vi "Device Test.vi"() -> ()   [LabVIEW 2011, in "Power Supply.lvclass"]
uses:
  Power Supply.lvclass
  Protection Limits.ctl
  Voltage Units.ctl
  Current Units.ctl
  Source Units.ctl
  Keithley 2400/Keithley 2400.lvclass
  Stanford Research PS350/Stanford Research PS350.lvclass
  Source Mode.ctl
panel:
  out "Source Value":dbl
  out "output":bool
  in  "Test":T1(ring)
  out "error out":errorcluster
  in  "Power Supply":enum16{"Keithley", "Stanford Research"}(ring)
  in  "Source Value Units":T2
  in  "Source Value":dbl=20.0
  in  "Limits":T3={"Voltage Limit"=100.0, "Voltage Limit Units"=enum."volts", "Current Limit"=1.0, "Current Limit Units"=enum."microamps", "Voltage Trip/Cmpl"=50.0, "Voltage Trip/Cmpl Units"=enum."volts", "Current Trip/Cmpl"=1.0, "Current Trip/Cmpl Units"=enum."microamps"}
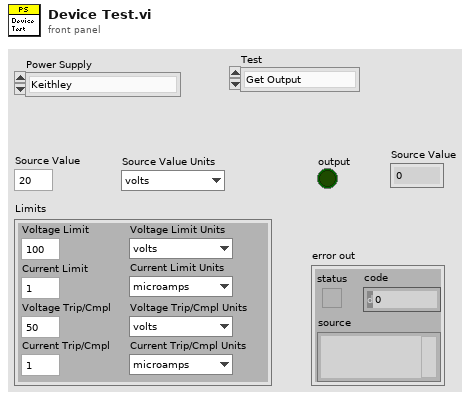
[diagram p1: front panel]
types:
  T1 = enum16{"Get Output", "Get Source Value", "Set Voltage"}
  T2 = typedef "Power Supply.lvclass/Source Units.ctl" = enum16{"volts", "millivolts", "microvolts", "amps", "milliamps", "microamps", "nanoamps"}
  T3 = typedef "Power Supply.lvclass/Protection Limits.ctl" = cluster{"Voltage Limit":dbl, "Voltage Limit Units":T4, "Current Limit":dbl, "Current Limit Units":T5, "Voltage Trip/Cmpl":dbl, "Voltage Trip/Cmpl Units":T4, "Current Trip/Cmpl":dbl, "Current Trip/Cmpl Units":T5}
  T4 = typedef "Power Supply.lvclass/Voltage Units.ctl" = enum16{"volts", "millivolts", "microvolts"}
  T5 = typedef "Power Supply.lvclass/Current Units.ctl" = enum16{"amps", "milliamps", "microamps", "nanoamps"}
  T6 = typedef "Power Supply.lvclass/Source Mode.ctl" = enum16{"Volts", "Current"}
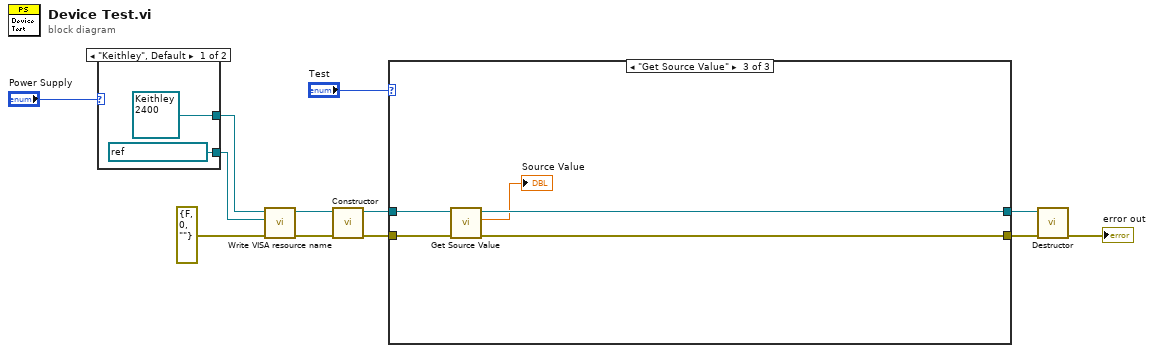
[diagram p0: block diagram]
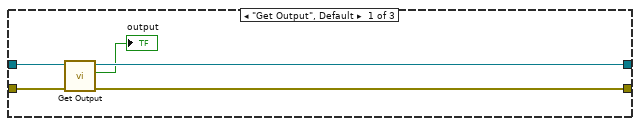
[diagram p2: hidden frame]
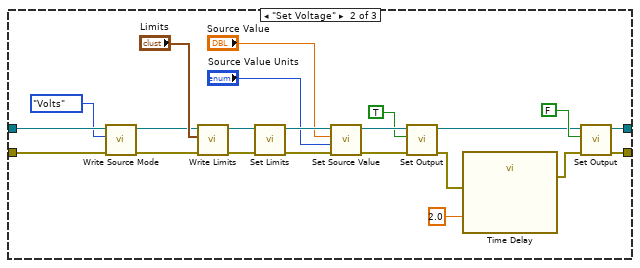
[diagram p3: hidden frame]
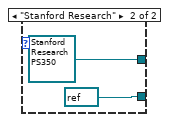
[diagram p4: hidden frame]
diagram:
  n1 = case shown="\"Keithley\", Default" "Power Supply" {
    tunnel: [refnum<class "Keithley 2400.lvclass"> refnum ("Keithley 2400.lvclass") refnum<class "Stanford Research PS350.lvclass"> refnum ("Stanford Research PS350.lvclass")] -> w4
    tunnel: [refnum<visa-resource-name> "Keithley_2400" ("VISA resource name") refnum<visa-resource-name> refnum ("VISA resource name")] -> w1
    frame "Keithley", Default {
    }
    frame "Stanford Research" {
    }
  }
  n2 = call-dynamic "Write VISA resource name.vi"("error in (no error)"=errorcluster {"status"=FALSE, "code"=0, "source"=""}, "VISA resource name"=w1, "Power Supply in"=w4) -> ("error out"=w2:errorcluster, "Power Supply out"=w3:refnum<class "Power Supply.lvclass">)  [unwired: 7 in]
  n3 = call-dynamic "Constructor.vi"("error in (no error)"=w2, "Power Supply in"=w3) -> ("error out"=w6:errorcluster, "Power Supply out"=w7:refnum<class "Power Supply.lvclass">)  [unwired: 7 in, 1 out]
  n4 = case shown="\"Get Source Value\"" "Test" {
    tunnel: [w21 w28 w46] -> w11
    tunnel: [w20 w27 w45] -> w10
    tunnel: w7 -> [w19 w26 w48]
    tunnel: w6 -> [w18 w25 w47]
    frame "Get Output", Default {
      n5 = call-dynamic "Get Output.vi"("error in (no error)"=w18, "Power Supply in"=w19) -> ("error out"=w20:errorcluster, "output"=→"output":bool, "Power Supply out"=w21:refnum<class "Power Supply.lvclass">)  [unwired: 7 in]
    }
    frame "Set Voltage" {
      n6 = call-dynamic "Write Source Mode.vi"("error in (no error)"=w25, "Source Mode"=Source_Mode."Volts", "Power Supply in"=w26) -> ("error out"=w23:errorcluster, "Power Supply out"=w24:refnum<class "Power Supply.lvclass">)  [unwired: 7 in]
      n7 = call-dynamic "Write Limits.vi"("error in (no error)"=w23, "Limits"="Limits", "Power Supply in"=w24) -> ("error out"=w41:errorcluster, "Power Supply out"=w42:refnum<class "Power Supply.lvclass">)  [unwired: 7 in]
      n8 = call-dynamic "Set Limits.vi"("error in (no error)"=w41, "Power Supply in"=w42) -> ("error out"=w39:errorcluster, "Power Supply out"=w40:refnum<class "Power Supply.lvclass">)  [unwired: 8 in]
      n9 = call-dynamic "Set Source Value.vi"("error in (no error)"=w39, "Source Value Units"="Source Value Units", "Source Value"="Source Value", "Power Supply in"=w40) -> ("error out"=w35:errorcluster, "Power Supply out"=w36:refnum<class "Power Supply.lvclass">)  [unwired: 6 in]
      n10 = call-dynamic "Set Output.vi"("error in (no error)"=w35, "Enable"=TRUE, "Power Supply in"=w36) -> ("error out"=w32:errorcluster, "Power Supply out"=w30:refnum<class "Power Supply.lvclass">)  [unwired: 7 in]
      n11 = call "Time Delay"("error in (no error)"=w32, "Delay Time (s)"=2.0) -> ("error out"=w29:errorcluster)  [unwired: 9 in]
      n12 = call-dynamic "Set Output.vi"("error in (no error)"=w29, "Enable"=FALSE, "Power Supply in"=w30) -> ("error out"=w27:errorcluster, "Power Supply out"=w28:refnum<class "Power Supply.lvclass">)  [unwired: 7 in]
    }
    frame "Get Source Value" {
      n13 = call-dynamic "Get Source Value.vi"("error in (no error)"=w47, "Power Supply in"=w48) -> ("error out"=w45:errorcluster, "Source Value"=→"Source Value":dbl, "Power Supply out"=w46:refnum<class "Power Supply.lvclass">)  [unwired: 6 in, 1 out]
    }
  }
  n14 = call-dynamic "Destructor.vi"("error in (no error)"=w10, "Power Supply in"=w11) -> ("error out"=→"error out":errorcluster)  [unwired: 8 in, 1 out]
